vi "set_all_pdos_state.vi"(11 "state":u8) -> ()   [LabVIEW 2011]
uses:
  canopen_dll_master.dll
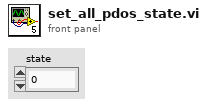
[diagram p1: front panel]
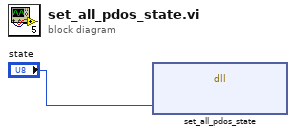
[diagram p0: block diagram]
diagram:
  n1 = dll-call lib="canopen_dll_master.dll" fn="set_all_pdos_state"("state"="state") -> ()  [unwired: 5 in, 2 out]
